vi "ConvertTextBasedCodeToLabVIEW_FindGenerics.vi"(11 "Classes":T1[](array[typedef])) -> (3 "ClassesOut":T1[](array[typedef]))   [LabVIEW 2020]
uses:
  <resource>/Framework/Providers/Open_GDS/ClassProviders/Common/String/GDSString_ClassDescriptionType.ctl
  <resource>/Framework/Providers/Open_GDS/ClassProviders/Common/String/GDSString_AccessScopeModifierType.ctl
  <resource>/Framework/Providers/Open_GDS/ClassProviders/Common/String/GDSString_ModifierType.ctl
  <resource>/Framework/Providers/Open_GDS/ClassProviders/Common/String/GDSString_MethodDescriptionType.ctl
  <resource>/Framework/Providers/Open_GDS/ClassProviders/Common/CommonVIs/CommonVIs_AttributeType.ctl
  <resource>/Framework/Providers/Open_GDS/ClassProviders/Common/CommonVIs/CommonVIs_AttributeDataType.ctl
  <resource>/Framework/Providers/Open_GDS/ClassProviders/Common/CommonVIs/CommonVIs_PropertyType.ctl
  <resource>/Framework/Providers/Open_GDS/ClassProviders/Common/String/GDSString_ClassParentType.ctl
  <resource>/Framework/Providers/Open_GDS/ClassProviders/Common/String/GDSString_ClassType.ctl
  <resource>/Framework/Providers/Open_GDS/ClassProviders/Common/String/GDSString_ClassOwnerType.ctl
  <resource>/Framework/Providers/Open_GDS/ClassProviders/Common/CommonVIs/CommonVIs_EnumType.ctl
  <resource>/Framework/Providers/Open_GDS/ClassProviders/Common/CommonVIs/CommonVIs_StructType.ctl
panel:
  out "Array":T13(array[cluster])
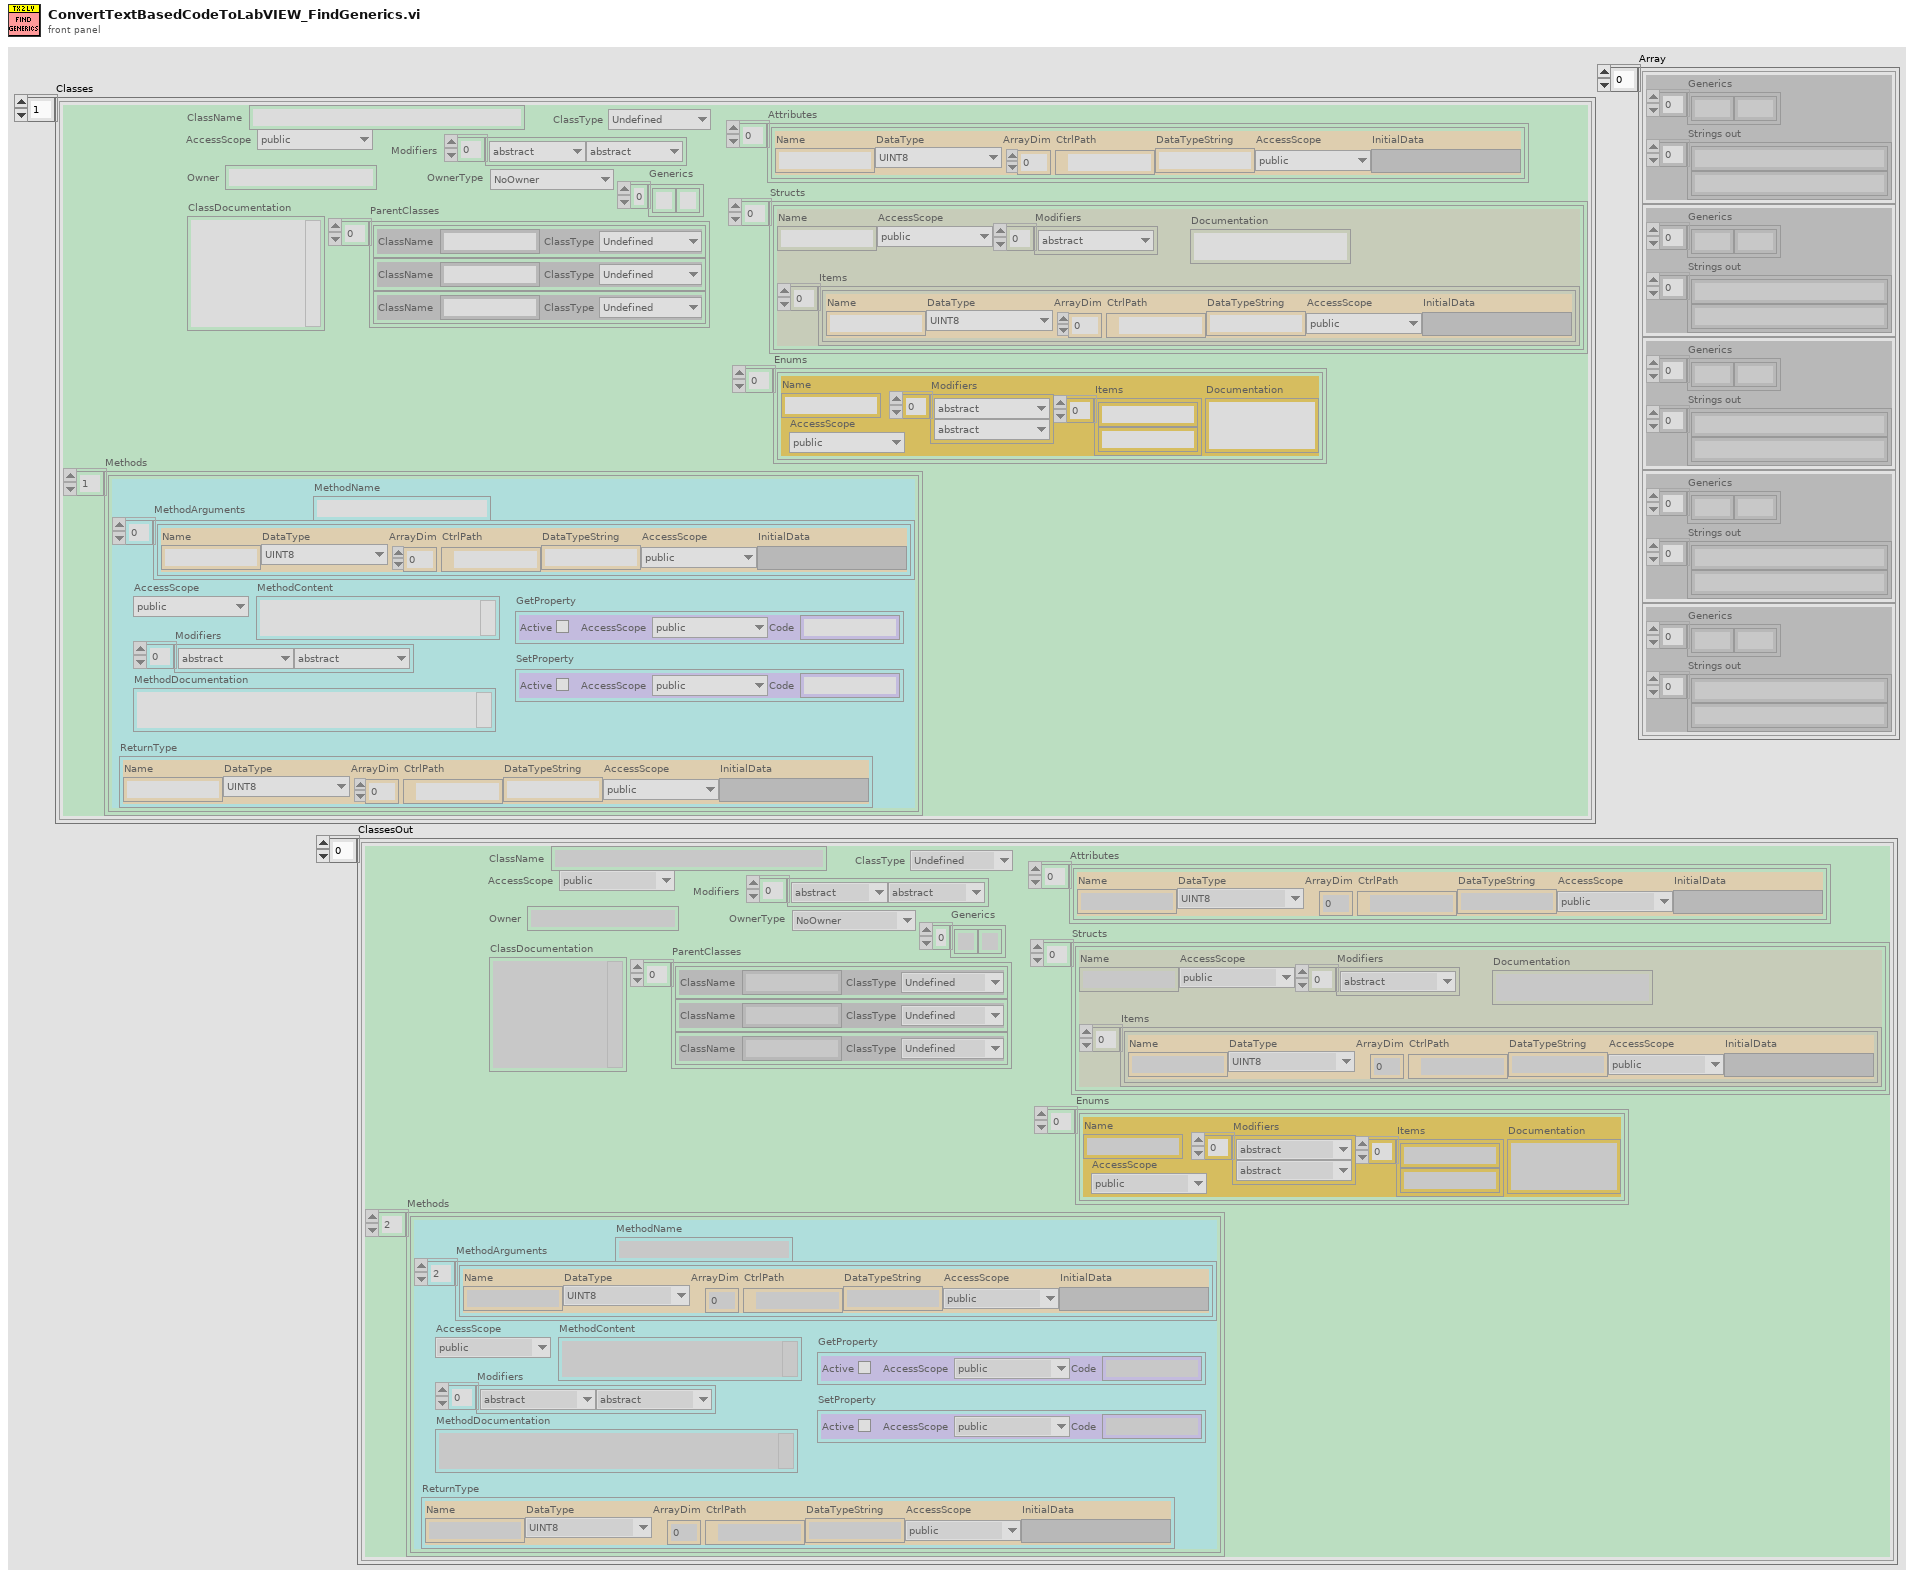
[diagram p1: front panel]
types:
  T1 = typedef "GDSString_ClassDescriptionType.ctl" = cluster{"ClassName":string, "AccessScope":T2, "Modifiers":T3[], "ClassDocumentation":string, "Methods":T4[], "ParentClasses":T8[], "ClassType":T9, "Owner":string, "OwnerType":T10, "Generics":string[], "Attributes":T5[], "Enums":T11[], "Structs":T12[]}
  T2 = typedef "GDSString_AccessScopeModifierType.ctl" = enum16{"public", "private", "protected", "internal"}
  T3 = typedef "GDSString_ModifierType.ctl" = enum16{"abstract", "static", "final", "synchronized", "strictfp", "async", "const", "event", "extern", "new", "native ", "override", "partial", "readonly", "sealed", "unsafe", "virtual", "volatile"}
  T4 = typedef "GDSString_MethodDescriptionType.ctl" = cluster{"ReturnType":T5, "MethodName":string, "AccessScope":T2, "Modifiers":T3[], "MethodDocumentation":string, "MethodContent":string, "MethodArguments":T5[], "GetProperty":T7, "SetProperty":T7}
  T5 = typedef "CommonVIs_AttributeType.ctl" = cluster{"Name":string, "DataType":T6, "ArrayDim":i32, "CtrlPath":path, "DataTypeString":string, "AccessScope":T2, "InitialData":variant}
  T6 = typedef "CommonVIs_AttributeDataType.ctl" = enum16{"UINT8", "INT8", "UINT16", "INT16", "UINT32", "INT32", "UINT64", "INT64", "SGL", "DBL", "EXT", "CSG", "CDB", "CXT", "TimeStamp", "STRING", "PATH", "BOOL", "ENUM", "RefNum", "VIRefNum", "LabVIEW Class", "Cluster", "Variant", "TypeDef", "Waveform", "LabVIEW Object", "Other", "void", "Set", "Map"}
  T7 = typedef "CommonVIs_PropertyType.ctl" = cluster{"Active":bool, "AccessScope":T2, "Code":string}
  T8 = typedef "GDSString_ClassParentType.ctl" = cluster{"ClassName":string, "ClassType":T9}
  T9 = typedef "GDSString_ClassType.ctl" = enum16{"Undefined", "Class", "Interface"}
  T10 = typedef "GDSString_ClassOwnerType.ctl" = enum16{"NoOwner", "Class", "Package/NameSpace"}
  T11 = typedef "CommonVIs_EnumType.ctl" = cluster{"Name":string, "AccessScope":T2, "Modifiers":T3[], "Items":string[], "Documentation":string}
  T12 = typedef "CommonVIs_StructType.ctl" = cluster{"Name":string, "AccessScope":T2, "Modifiers":T3[], "Items":T5[], "Documentation":string}
  T13 = cluster{"Generics":string[], "Strings out":string[]}[]
  T14 = cluster{"Generics":string[], "Strings out":string[]}
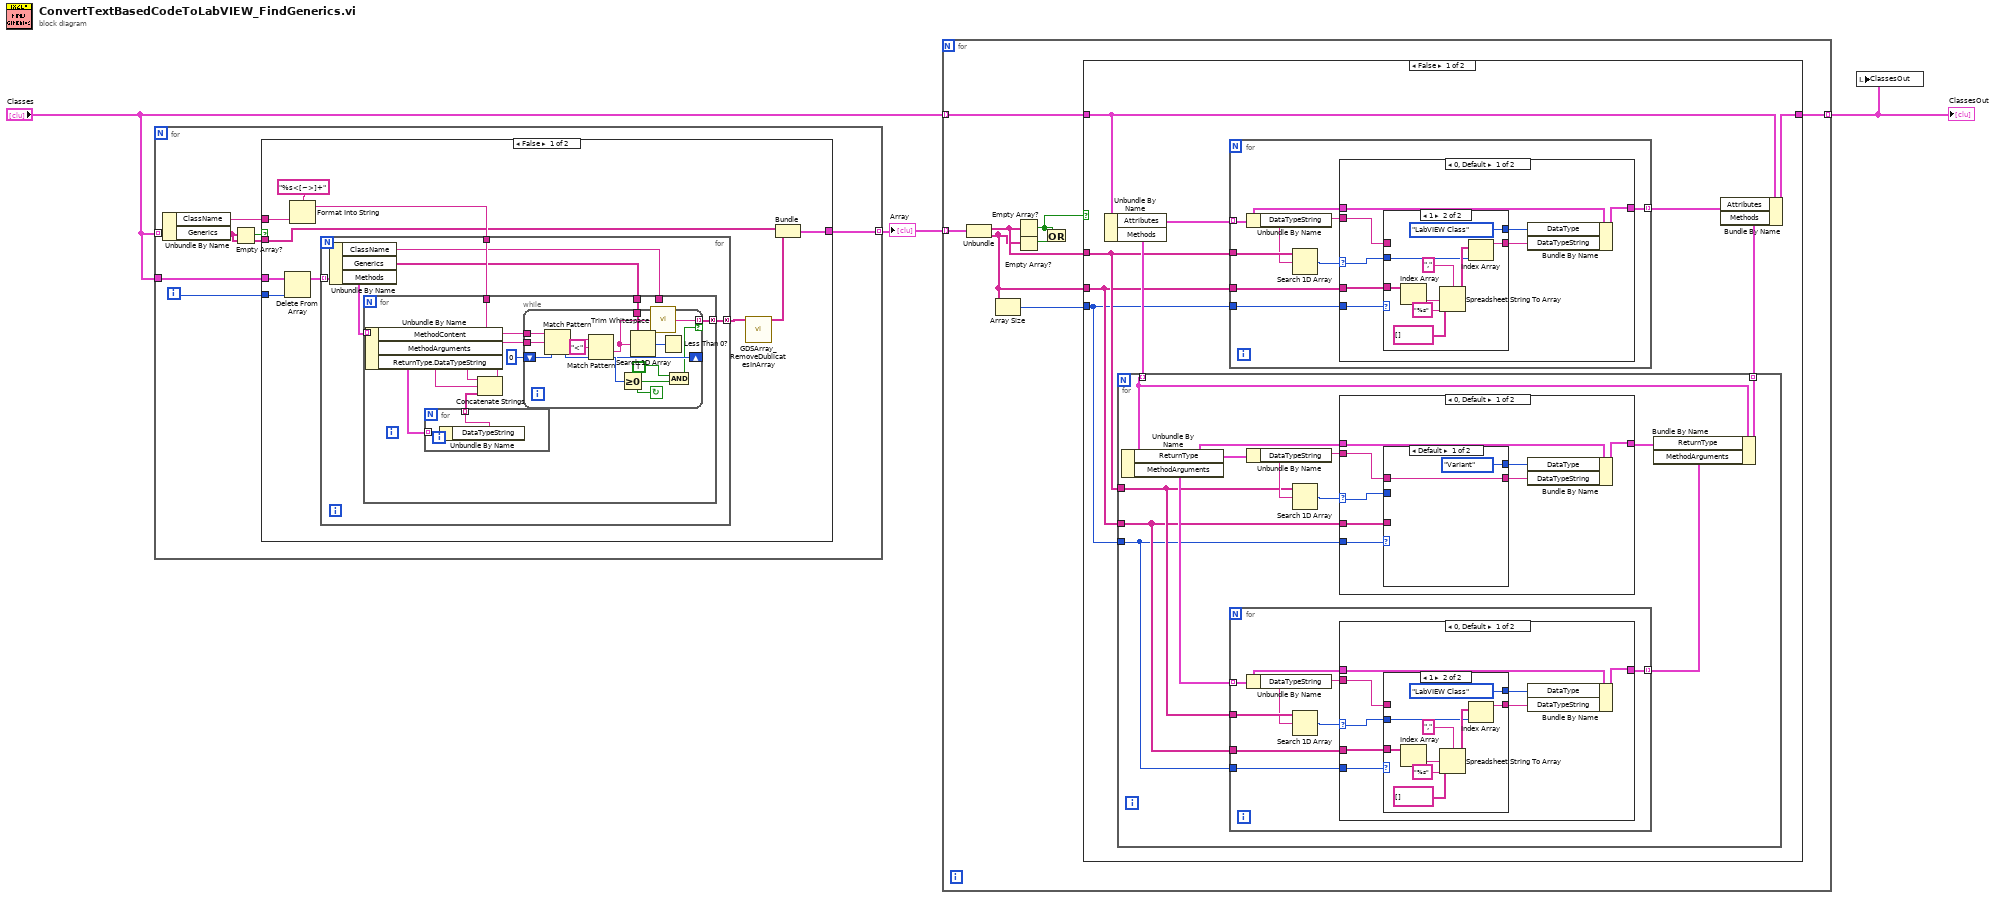
[diagram p0: block diagram]
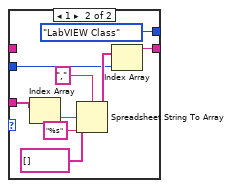
[diagram p2: hidden frame]
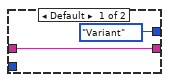
[diagram p4: hidden frame]
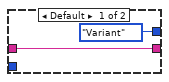
[diagram p6: hidden frame]
diagram:
  n1 = for {
    tunnel: "Classes" -> [w10] mode=indexing
    tunnel: "Classes" -> [w8]
    tunnel: [w4] -> w1 mode=indexing
    i -> [w7]
    n2 = Unbundle By Name(w10) -> ("ClassName"=w6:string, "Generics"=w5:string[])
    n3 = Empty Array?(array=w5) -> (empty?=w9:bool)
    n4 = case shown="False" w9 {
      tunnel: w8 -> [w20 _]
      tunnel: w7 -> [w19 _]
      tunnel: w6 -> [w17 _]
      tunnel: w5 -> [w13 _]
      tunnel: [w11 _] -> w4
      frame False {
        n5 = Delete From Array(array=w20, index=w19) -> (array with subset deleted=w18:T1[])  [unwired: 1 in, 1 out]
        n6 = Format Into String(format string="%s<[~>]+", w17) -> (resulting string=w15:string)  [unwired: 2 in, 1 out]
        n7 = for {
          tunnel: w18 -> [w26] mode=indexing
          tunnel: w15 -> [w24]
          tunnel: [w22] -> w14 mode=concatenating
          n8 = Unbundle By Name(w26) -> ("ClassName"=w21:string, "Generics"=w23:string[], "Methods"=w25:T4[])
          n9 = for {
            tunnel: w25 -> [w36] mode=indexing
            tunnel: w24 -> [w35]
            tunnel: w23 -> [w34]
            tunnel: [w33] -> w22 mode=concatenating
            tunnel: w21 -> [_]
            n10 = Unbundle By Name(w36) -> ("MethodContent"=w30:string, "MethodArguments"=w32:T5[], "ReturnType.DataTypeString"=w27:string)
            n11 = for {
              tunnel: w32 -> [w52] mode=indexing
              tunnel: [w51] -> w31 mode=indexing
              n12 = Unbundle By Name(w52) -> ("DataTypeString"=w51:string)
            }
            n13 = Concatenate Strings(w30, w27, w31) -> (w29:string)
            n14 = while {
              tunnel: w35 -> [w50]
              tunnel: w34 -> [w47]
              tunnel: [w38] -> w33 mode=indexing if=w39
              tunnel: w29 -> [w43]
              shift-right: [w41] -> _
              shift-left: 0 ("offset past match") -> [w42]
              stop <- w40 continue-if-true
              n15 = Match Pattern(string=w43, regular expression=w50, offset (0)=w42) -> (match substring=w49:string, offset past match=w41:i32)  [unwired: 2 out]
              n16 = Match Pattern(string=w49, regular expression="<") -> (after substring=w45:string, offset past match=w44:i32)  [unwired: 1 in, 2 out]
              n17 = Greater Or Equal To 0?(x=w44) -> (x >= 0?=w40:bool)
              n18 = Search 1D Array(1D array=w47, element=w45) -> (index of element=w46:i32)  [unwired: 1 in]
              n19 = call <vilib>:"Trim Whitespace.vi"("string"=w45) -> ("trimmed string"=w38:string)  [unwired: 1 in]
              n20 = Less Than 0?(x=w46) -> ()  [unwired: 1 out]
              n21 = And(x=TRUE, y=w40) -> (x .and. y?=w39:bool)
            }
          }
        }
        n22 = call <resource>:"GDSArray_RemoveDublicatesInArray.vi"("Strings in"=w14) -> ("Strings out"=w12:string[])  [unwired: 16 in, 2 out]
        n23 = Bundle("Generics"=w13, "Strings out"=w12) -> (w11:T14)  [unwired: 1 in]
      }
      frame True {
      }
    }
  }
  "Array" <- w1
  n24 = for {
    tunnel: "Classes" -> [w58] mode=indexing
    tunnel: w1 -> [w60] mode=indexing
    tunnel: [w57] -> w3 mode=indexing
    n25 = Unbundle(w60) -> ("Generics"=w56:string[], "Strings out"=w55:string[])
    n26 = Array Size(array=w55) -> (size(s)=w54:i32)
    n27 = Empty Array?(array=w56) -> (empty?=w53:bool)
    n28 = Empty Array?(array=w55) -> (empty?=w59:bool)
    n29 = Or(x=w53, y=w59) -> ()  [unwired: 1 out]
    n30 = case shown="False" w53 {
      tunnel: w58 -> [w69 w155]
      tunnel: [w66 w155] -> w57
      tunnel: w56 -> [w64 _]
      tunnel: w55 -> [w63 _]
      tunnel: w54 -> [w62 _]
      frame False {
        n31 = Unbundle By Name(w69) -> ("Attributes"=w68:T5[], "Methods"=w65:T4[])
        n32 = for {
          tunnel: w65 -> [w73] mode=indexing
          tunnel: w64 -> [w76]
          tunnel: w63 -> [w75]
          tunnel: w62 -> [w74]
          tunnel: [w70] -> w61 mode=indexing
          n33 = Unbundle By Name(w73) -> ("ReturnType"=w77:T5, "MethodArguments"=w80:T5[])
          n34 = for {
            tunnel: w80 -> [w105] mode=indexing
            tunnel: w76 -> [w107]
            tunnel: [w104] -> w71 mode=indexing
            tunnel: w75 -> [w102]
            tunnel: w74 -> [w101]
            n35 = Unbundle By Name(w105) -> ("DataTypeString"=w103:string)
            n36 = Search 1D Array(1D array=w107, element=w103) -> (index of element=w106:i32)  [unwired: 1 in]
            n37 = case shown="0, Default" w106 {
              selector: w106 -> [w108 _]
              tunnel: w105 -> [w115 w127]
              tunnel: [w114 w127] -> w104
              tunnel: w103 -> [w112 _]
              tunnel: w102 -> [w109 _]
              tunnel: w101 -> [w110 _]
              frame 0, Default {
                n38 = case shown="1" w110 {
                  tunnel: [CommonVIs_AttributeDataType."Variant" ("DataType") CommonVIs_AttributeDataType."LabVIEW Class" ("DataType")] -> w113
                  tunnel: w112 -> [w116 _]
                  tunnel: [w116 w119] -> w111
                  tunnel: w109 -> [_ w125]
                  tunnel: w108 -> [_ w118]
                  frame Default {
                  }
                  frame 1 {
                    n39 = Index Array(array=w125) -> (element=w124:string)  [unwired: 1 in]
                    n40 = Spreadsheet String To Array(delimiter (Tab)=",", format string="%s", spreadsheet string=w124, array type (2D Dbl)=string[] []) -> (array=w120:string[])
                    n41 = Index Array(array=w120, index=w118) -> (element=w119:string)
                  }
                }
                n42 = Bundle By Name(cluster=w115, "DataType"=w113, "DataTypeString"=w111) -> (w114:T5)
              }
              frame -1 {
              }
            }
          }
          n43 = Unbundle By Name(w77) -> ("DataTypeString"=w78:string)
          n44 = Search 1D Array(1D array=w76, element=w78) -> (index of element=w79:i32)  [unwired: 1 in]
          n45 = case shown="0, Default" w79 {
            selector: w79 -> [w81 _]
            tunnel: w77 -> [w88 w100]
            tunnel: [w87 w100] -> w72
            tunnel: w78 -> [w85 _]
            tunnel: w75 -> [w82 _]
            tunnel: w74 -> [w83 _]
            frame 0, Default {
              n46 = case shown="Default" w83 {
                tunnel: [CommonVIs_AttributeDataType."Variant" ("DataType") CommonVIs_AttributeDataType."LabVIEW Class" ("DataType")] -> w86
                tunnel: w85 -> [w89 _]
                tunnel: [w89 w92] -> w84
                tunnel: w82 -> [_ w98]
                tunnel: w81 -> [_ w91]
                frame Default {
                }
                frame 1 {
                  n47 = Index Array(array=w98) -> (element=w97:string)  [unwired: 1 in]
                  n48 = Spreadsheet String To Array(delimiter (Tab)=",", format string="%s", spreadsheet string=w97, array type (2D Dbl)=string[] []) -> (array=w93:string[])
                  n49 = Index Array(array=w93, index=w91) -> (element=w92:string)
                }
              }
              n50 = Bundle By Name(cluster=w88, "DataType"=w86, "DataTypeString"=w84) -> (w87:T5)
            }
            frame -1 {
            }
          }
          n51 = Bundle By Name(cluster=w73, "ReturnType"=w72, "MethodArguments"=w71) -> (w70:T4)
        }
        n52 = for {
          tunnel: w68 -> [w132] mode=indexing
          tunnel: w64 -> [w134]
          tunnel: [w131] -> w67 mode=indexing
          tunnel: w63 -> [w129]
          tunnel: w62 -> [w128]
          n53 = Unbundle By Name(w132) -> ("DataTypeString"=w130:string)
          n54 = Search 1D Array(1D array=w134, element=w130) -> (index of element=w133:i32)  [unwired: 1 in]
          n55 = case shown="0, Default" w133 {
            selector: w133 -> [w135 _]
            tunnel: w132 -> [w142 w154]
            tunnel: [w141 w154] -> w131
            tunnel: w130 -> [w139 _]
            tunnel: w129 -> [w136 _]
            tunnel: w128 -> [w137 _]
            frame 0, Default {
              n56 = case shown="1" w137 {
                tunnel: [CommonVIs_AttributeDataType."Variant" ("DataType") CommonVIs_AttributeDataType."LabVIEW Class" ("DataType")] -> w140
                tunnel: w139 -> [w143 _]
                tunnel: [w143 w146] -> w138
                tunnel: w136 -> [_ w152]
                tunnel: w135 -> [_ w145]
                frame Default {
                }
                frame 1 {
                  n57 = Index Array(array=w152) -> (element=w151:string)  [unwired: 1 in]
                  n58 = Spreadsheet String To Array(delimiter (Tab)=",", format string="%s", spreadsheet string=w151, array type (2D Dbl)=string[] []) -> (array=w147:string[])
                  n59 = Index Array(array=w147, index=w145) -> (element=w146:string)
                }
              }
              n60 = Bundle By Name(cluster=w142, "DataType"=w140, "DataTypeString"=w138) -> (w141:T5)
            }
            frame -1 {
            }
          }
        }
        n61 = Bundle By Name(cluster=w69, "Attributes"=w67, "Methods"=w61) -> (w66:T1)
      }
      frame True {
      }
    }
  }
  "ClassesOut" <- w3
  n62 = local write "ClassesOut"(w3) -> ()
